vi "Create VariantBufferMap.vi"(8 "error in":errorcluster, 11 "bufSize":i32) -> (0 "error out":errorcluster, 3 "BufferMap":refnum<data-value>)   [LabVIEW 2013, in "CircularBuffer.lvlib" / "VariantBufferMap.lvclass"]
doc: "This VI creates a ring buffer of set size. This buffer is created in one place in the memory and is then accessed via pointer/reference.\n\nThe Data Type input is required because it defines the place in the memory to correct size thus removing the need for memory reallocation."
uses:
  VariantBufferMap.lvclass
  VariantBuffer/VariantBuffer.lvclass
  VariantBufferMap.lvclass/VariantBufferMap.ctl
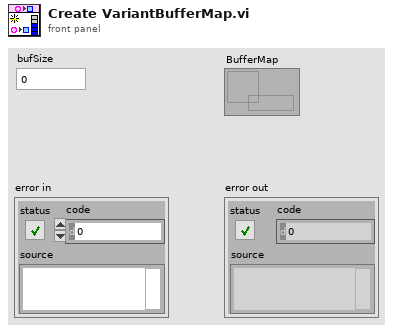
[diagram p1: front panel]
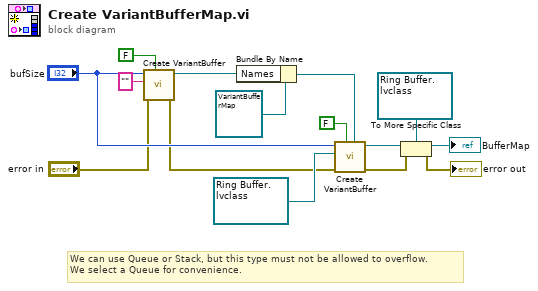
[diagram p0: block diagram]
diagram:
  # "We can use Queue or Stack, but this type must not be allowed to overflow.\nWe select a Queue for convenience."
  n1 = call "Create VariantBuffer.vi"("Allow Overflow? (T)"=FALSE, "error in"="error in", "default"="", "bufSize"="bufSize") -> ("error out"=w4:errorcluster, "Buffer"=w11:refnum<data-value>)  [unwired: 6 in]
  n2 = Bundle By Name(cluster=refnum<class "VariantBufferMap.lvclass"> refnum ("Ring Buffer.lvclass"), "Names"=w11) -> (w1:refnum<class "VariantBufferMap.lvclass">)
  n3 = call "Create VariantBuffer.vi"("Buffer"=w1, "Allow Overflow? (T)"=FALSE, "error in"=w4, "default"=refnum<data-value> refnum ("Buffer"), "bufSize"="bufSize") -> ("error out"=w6:errorcluster, "Buffer"=w10:refnum<data-value>)  [unwired: 5 in]
  n4 = To More Specific Class(target class=refnum<data-value> refnum ("BufferMap"), reference=w10, error in=w6) -> (specific class reference=→"BufferMap":refnum<data-value>, error out=→"error out":errorcluster)
